vi "plot_waypoints.vi"(8 "Mission Waypoint?":bool, 9 "MapDistanceInfo":T1 {"Top Left Pixel UTM"."North" format="%#_10f"; "Top Left Pixel UTM"."East" format="%#_8f"; "Bottom Right Pixel UTM"."North" format="%#_10f"; "Bottom Right Pixel UTM"."East" format="%#_8f"}, 10 "Waypoint Array":refnum<class "Waypoint.lvclass">[](array[class]), 11 "Map in":T3) -> (2 "WP Outside Img":bool, 3 "Map Out":T3)   [LabVIEW 2013]
uses:
  <vilib>/vision/Image Controls.llb/IMAQ Image.ctl
  TypeDef/map_metadata.ctl
  cRIO_Code/Data/TypeDefs/UTM Location.ctl
  cRIO_Code/Logic/Classes/Waypoint/Waypoint.lvclass
panel:
  out "MapDistanceInfo OUT":T1 {"Top Left Pixel UTM"."North" format="%#_10f"; "Top Left Pixel UTM"."East" format="%#_8f"; "Bottom Right Pixel UTM"."North" format="%#_10f"; "Bottom Right Pixel UTM"."East" format="%#_8f"}
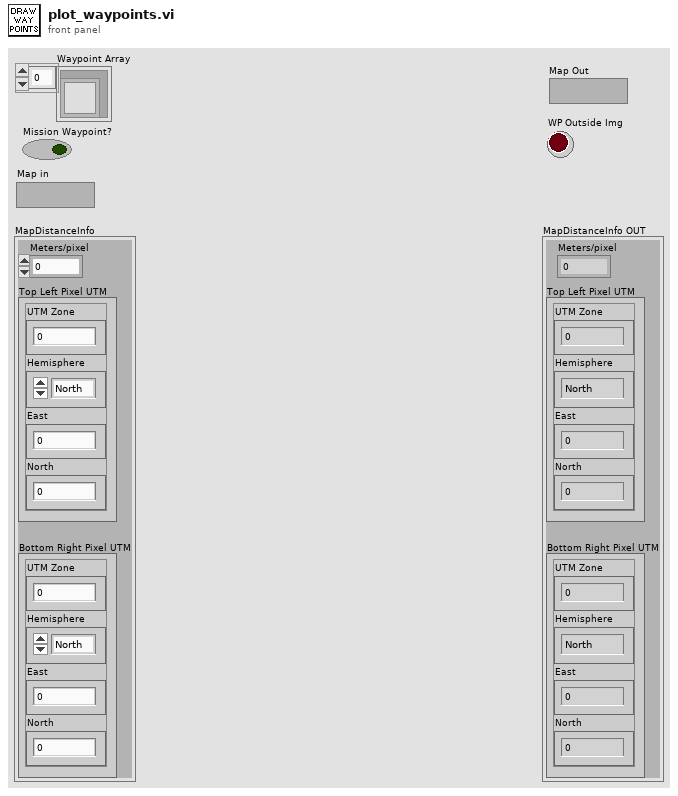
[diagram p1: front panel]
types:
  T1 = typedef "map_metadata.ctl" = cluster{"Meters/pixel":dbl, "Top Left Pixel UTM":T2, "Bottom Right Pixel UTM":T2}
  T2 = typedef "UTM Location.ctl" = cluster{"UTM Zone":dbl, "Hemisphere":enum16{"North", "South"}, "East":dbl, "North":dbl}
  T3 = typedef "IMAQ Image.ctl" = refnum<image>
  T4 = typedef "waypoint_icon_references.ctl" = cluster{"Mission Waypoint Icon":T3, "Sailing Point Icon":T3, "Mission Waypoint Done Icon":T3, "Sailing Point Done Icon":T3, "Next Mission Waypoint Icon":T3, "Next Sailing Point Icon":T3}
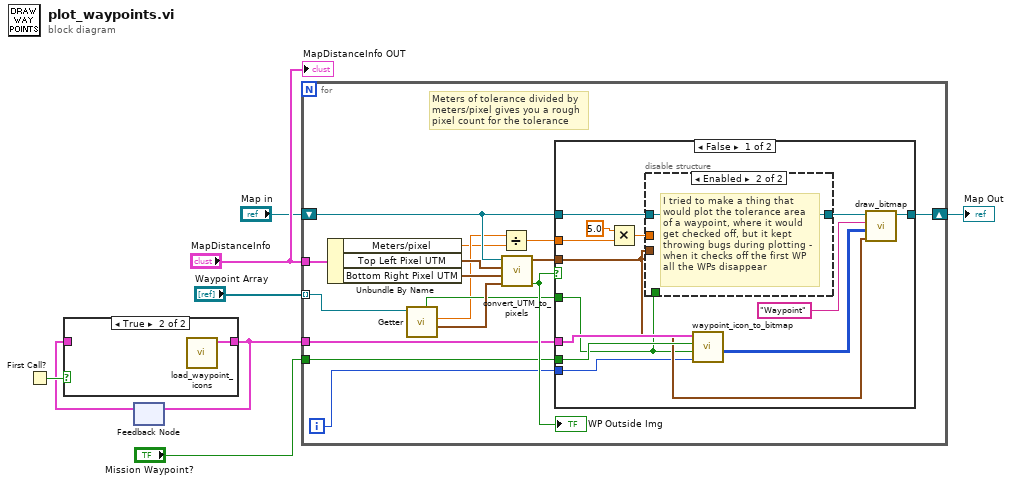
[diagram p0: block diagram]
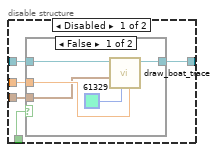
[diagram p3: hidden frame]
diagram:
  n1 = First Call?() -> (First Call?: T/F=w4:bool)
  n2 = feedback #1() -> (w3:T4)  [unwired: 1 in]
  n3 = case shown="True" w4 {
    tunnel: [w9 w10] -> w2
    tunnel: w3 -> [w9 _]
    frame False {
      # "image already loaded"
    }
    frame True {
      n4 = call "load_waypoint_icons.vi"() -> ("Waypoint Icon Reference"=w10:T4)  [unwired: 11 in]
    }
  }
  n5 = feedback-in #1(w2) -> ()
  n6 = for {
    tunnel: "MapDistanceInfo" -> [w23]
    shift-right: [w26] -> w8
    shift-left: "Map in" -> [w20]
    tunnel: "Waypoint Array" -> [w19] mode=indexing
    tunnel: w2 -> [w17]
    tunnel: "Mission Waypoint?" -> [w16]
    i -> [w11]
    # "Meters of tolerance divided by meters/pixel gives you a rough pixel count for the tolerance"
    n7 = Unbundle By Name(w23) -> ("Meters/pixel"=w13:dbl, "Top Left Pixel UTM"=w22:T2, "Bottom Right Pixel UTM"=w21:T2)
    n8 = call "Getter.vi"("Waypoint In"=w19) -> ("Coords"=w18:T2, "Tolerance (meters?)"=w14:dbl, "Done?"=w15:bool)  [unwired: 6 in, 2 out]
    n9 = Divide(x=w14, y=w13) -> (x/y=w12:dbl)
    n10 = call "convert_UTM_to_pixels.vi"("UTM position of Boat"=w18, "Bottom Right Pixel UTM"=w21, "Top Left Pixel UTM"=w22, "Map in"=w20) -> ("Boat Outside Img"=w25:bool, "Position"=w24:cluster{"X":i32, "Y":i32})  [unwired: 6 in]
    "WP Outside Img" <- w25
    n11 = case shown="False" w25 {
      tunnel: [w31 w52] -> w26
      tunnel: w20 -> [w36 w52]
      tunnel: w24 -> [w30 _]
      tunnel: w17 -> [w38 _]
      tunnel: w16 -> [w37 _]
      tunnel: w15 -> [w29 _]
      tunnel: w12 -> [w33 _]
      tunnel: w11 -> [w27 _]
      frame False {
        n12 = Multiply(x=5.0, y=w33) -> (x*y=w34:dbl)
        n13 = disable-structure shown="Enabled" {
          disable-tunnel: w36 -> [w44 w51]
          disable-tunnel: [w43 w51] -> w35
          disable-tunnel: w34 -> [w42 _]
          disable-tunnel: w30 -> [w41 _]
          disable-tunnel: w29 -> [w40 _]
          frame Disabled {
            n14 = case shown="False" w40 {
              tunnel: w44 -> [w49 w50]
              tunnel: [w48 w50] -> w43
              tunnel: w42 -> [w47 _]
              tunnel: w41 -> [w46 _]
              frame False {
                n15 = call "draw_boat_trace.vi"("Radius (px)"=w47, "circle color"=u32 61329, "Position"=w46, "Image In"=w49) -> ("Image Out"=w48:T3)  [unwired: 7 in]
              }
              frame True {
              }
            }
          }
          frame Enabled {
            # "I tried to make a thing that would plot the tolerance area of a waypoint, where it would get checked off, but it kept throwing bugs during plotting - when it checks off the first WP all the WPs disappear"
          }
        }
        n16 = call "waypoint_icon_to_bitmap.vi"("Index"=w27, "Done?"=w29, "Mission Waypoint?"=w37, "Waypoint Icon References"=w38) -> ("Icon Bitmap Out"=w28:u32[][])  [unwired: 6 in, 1 out]
        n17 = call "draw_bitmap.vi"("Position"=w30, "Boat Bitmap"=w28, "Group"="Waypoint", "Image In"=w35) -> ("Image Out"=w31:T3)  [unwired: 3 out]
      }
      frame True {
        # "don't draw if point outside image. Why not? lol"
      }
    }
  }
  "Map Out" <- w8
  "MapDistanceInfo OUT" <- "MapDistanceInfo"
